vi "stop vis.vi"() -> (0 "Abort error":errorcluster)   [LabVIEW 2016, in "main.lvlib"]
doc: "This vi stops each vi for the main control vi subpanel"
uses:
  main.lvlib
  Beamline sections/High Energy End/High energy.lvlib
  Beamline sections/R30/R30.lvlib
  Beamline sections/Transmission/Transmission.lvlib
  Beamline sections/Low Energy End/Low energy.lvlib
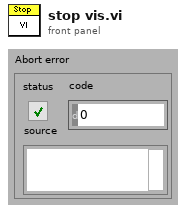
[diagram p1: front panel]
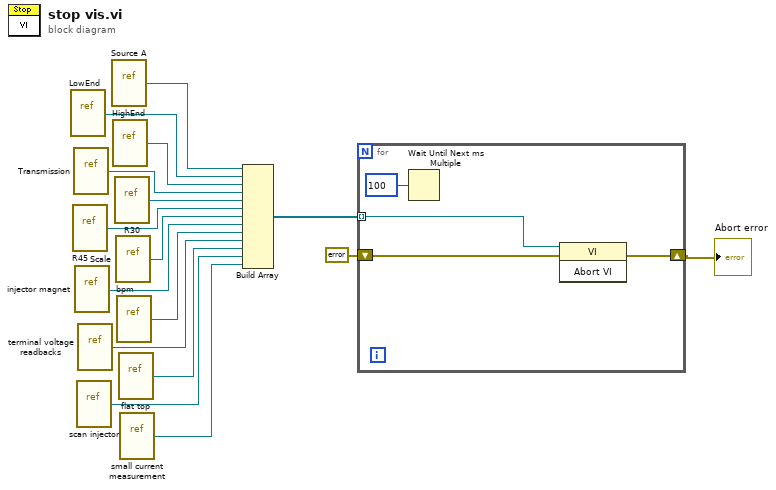
[diagram p0: block diagram]
diagram:
  n1 = vi-ref "LowEnd.vi"() -> (w12:refnum<vi>)
  n2 = vi-ref "R45.vi"() -> (w16:refnum<vi>)
  n3 = vi-ref "Transmission.vi"() -> (w14:refnum<vi>)
  n4 = vi-ref "injector magnet.vi"() -> (w7:refnum<vi>)
  n5 = vi-ref "scan injector.vi"() -> (w3:refnum<vi>)
  n6 = vi-ref "terminal voltage readbacks.vi"() -> (w5:refnum<vi>)
  n7 = vi-ref "Source A.vi"() -> (w11:refnum<vi>)
  n8 = vi-ref "HighEnd.vi"() -> (w13:refnum<vi>)
  n9 = vi-ref "R30.vi"() -> (w15:refnum<vi>)
  n10 = vi-ref "Scale.vi"() -> (w8:refnum<vi>)
  n11 = vi-ref "bpm.vi"() -> (w6:refnum<vi>)
  n12 = vi-ref "flat top.vi"() -> (w4:refnum<vi>)
  n13 = vi-ref "small current measurement.vi"() -> (w2:refnum<vi>)
  n14 = Build Array(w11, w12, w13, w14, w15, w16, w8, w7, w6, w5, w4, w3, w2) -> (w10:refnum<vi>[])
  n15 = for {
    shift-right: [w19] -> w9
    shift-left: errorcluster {"status"=FALSE, "code"=0, "source"=""} ("error out") -> [w18]
    tunnel: w10 -> [w17] mode=indexing
    n16 = Wait Until Next ms Multiple(millisecond multiple=u32 100) -> ()  [unwired: 1 out]
    n17 = invoke class="VI" method="Abort VI"(reference=w17, error in=w18) -> (error out=w19:errorcluster)  [unwired: 1 in, 2 out]
  }
  "Abort error" <- w9
